vi "Write Page Labels Visible.vi"(5 "Page Labels Visible":bool, 9 "Tab in":refnum<class "Tab.lvclass">) -> (3 "Tab out":refnum<class "Tab.lvclass">)   [LabVIEW 2014, in "Tab.lvclass"]
uses:
  Tab.lvclass
  Tab.lvclass/Tab.ctl
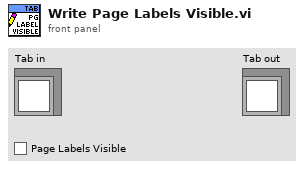
[diagram p1: front panel]
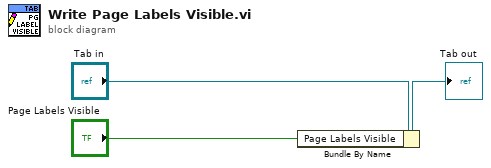
[diagram p0: block diagram]
diagram:
  n1 = Bundle By Name(cluster="Tab in", "Page Labels Visible"="Page Labels Visible") -> (→"Tab out":refnum<class "Tab.lvclass">)
